vi "get_positioning_cursors.vi"(8 "error in (no error)":errorcluster, 11 "ColorOverlay in":refnum<class "ColorOverlay.lvclass">) -> (0 "error out":errorcluster, 3 "ColorOverlay out":refnum<class "ColorOverlay.lvclass">)   [LabVIEW 2010, in "ColorOverlay.lvclass"]
uses:
  ColorOverlay.lvclass
  cursor_cluster.ctl
  ColorOverlay.lvclass/ColorOverlay.ctl
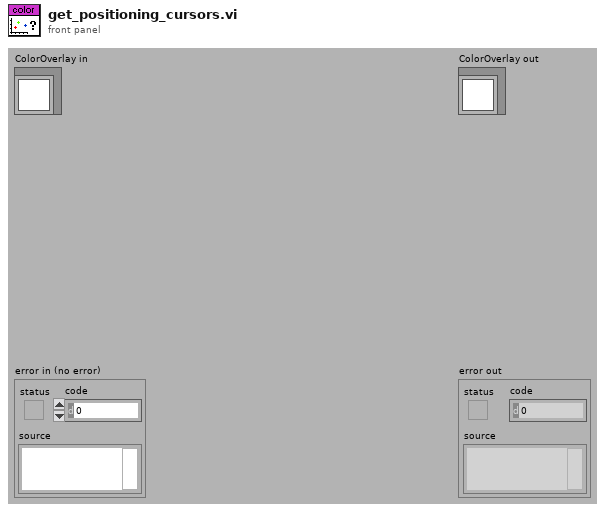
[diagram p1: front panel]
types:
  T1 = typedef "ColorOverlay.lvclass/cursor_cluster.ctl" = cluster{"cursor position":dbl[]}
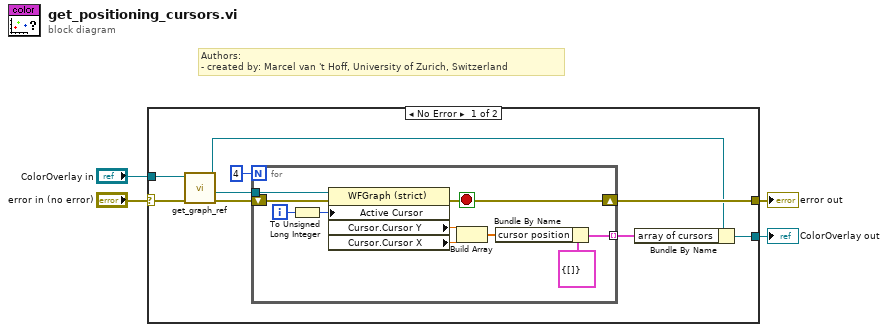
[diagram p0: block diagram]
diagram:
  # "Authors: \n- created by: Marcel van 't Hoff, University of Zurich, Switzerland"
  n1 = case shown="No Error" "error in (no error)" {
    selector: "error in (no error)" -> [w8 w25]
    tunnel: [w7 w25] -> w3
    tunnel: [w9 w24] -> w1
    tunnel: "ColorOverlay in" -> [w13 w24]
    frame No Error {
      n2 = call-dynamic "get_graph_ref.vi"("error in (no error)"=w8, "ColorOverlay in"=w13) -> ("error out"=w11:errorcluster, "graph ref"=w12:refnum<vi>, "ColorOverlay out"=w6:refnum<class "ColorOverlay.lvclass">)  [unwired: 7 in]
      n3 = for {
        N: 4 -> [_]
        tunnel: w12 -> [w23]
        shift-right: [w19] -> w7
        shift-left: w11 -> [w22]
        tunnel: [w15] -> w5 mode=indexing
        i -> [w21]
        stop <- w19 stop-if-true
        n4 = To Unsigned Long Integer(number=w21) -> (unsigned 32bit integer=w20:u32)
        n5 = property class="WFGraph (strict)"(reference=w23, error in=w22, "Active Cursor"=w20) -> (error out=w19:errorcluster, "Cursor.Cursor Y"=w18:dbl, "Cursor.Cursor X"=w17:dbl)  [unwired: 1 out]
        n6 = Build Array(w18, w17) -> (w16:dbl[])
        n7 = Bundle By Name(cluster=T1 {"cursor position"=[]} ("cursor positions"), "cursor position"=w16) -> (w15:T1)
      }
      n8 = Bundle By Name(cluster=w6, "array of cursors"=w5) -> (w9:refnum<class "ColorOverlay.lvclass">)
    }
    frame Error {
    }
  }
  "error out" <- w3
  "ColorOverlay out" <- w1
